vi "peak comb -- interpolate V1.vi"(6 "all peaks exp":i32[](array[numeric])=[564, 649, 987, 1133, 1214, 1585, 1763, 1823, 1880, 1899, 2032, 2138, 2221, 2270, 2350, 2456, 2580, 2634, 2831, 2960, 2965, 3131, 3328, 3469, 3553, 0, 3615, 3734, 0, 0, 0, 4236, 4300, 4331], 8 "Gamma":dbl, 11 "freq":dbl) -> (3 "Numeric":dbl)   [LabVIEW 2010]
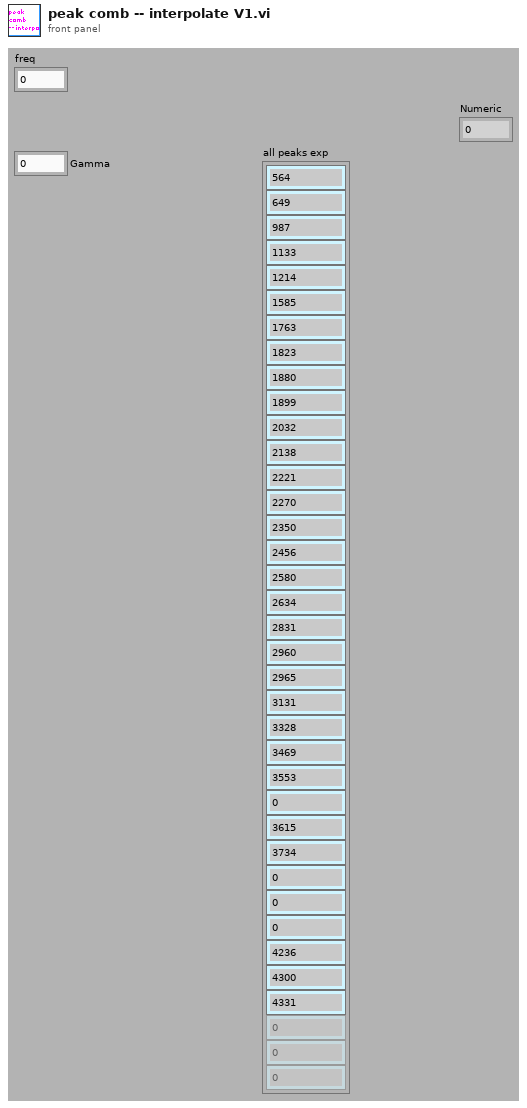
[diagram p1: front panel]
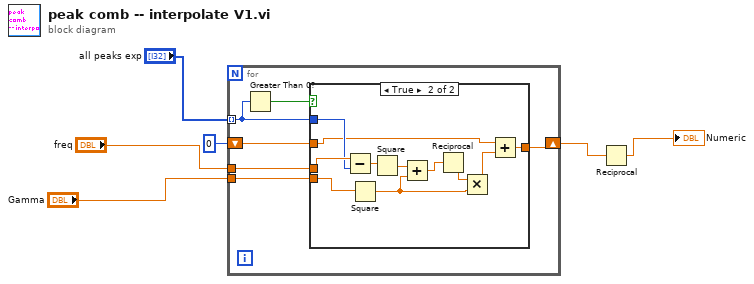
[diagram p0: block diagram]
diagram:
  n1 = for {
    tunnel: "all peaks exp" -> [w8] mode=indexing
    tunnel: "freq" -> [w12]
    tunnel: "Gamma" -> [w11]
    shift-right: [w9] -> w2
    shift-left: 0 -> [w10]
    n2 = Greater Than 0?(x=w8) -> (x > 0?=w7:bool)
    n3 = case shown="True" w7 {
      tunnel: w12 -> [_ w24]
      tunnel: w8 -> [_ w23]
      tunnel: w11 -> [_ w20]
      tunnel: w10 -> [w13 w19]
      tunnel: [w13 w18] -> w9
      frame False {
      }
      frame True {
        n4 = Subtract(x=w24, y=w23) -> (x-y=w22:dbl)
        n5 = Square(x=w20) -> (x^2=w15:dbl)
        n6 = Square(x=w22) -> (x^2=w21:dbl)
        n7 = Add(x=w21, y=w15) -> (x+y=w17:dbl)
        n8 = Reciprocal(x=w17) -> (1/x=w16:dbl)
        n9 = Multiply(x=w16, y=w15) -> (x*y=w14:dbl)
        n10 = Add(x=w19, y=w14) -> (x+y=w18:dbl)
      }
    }
  }
  n11 = Reciprocal(x=w2) -> (1/x=→"Numeric":dbl)
